vi "Compute SHA256 (byte array).vi"(10 "data in":u8[](array[numeric])) -> (2 "digest":u8[](array[numeric]) format="%02x")   [LabVIEW 2013, in "NI_SHA-256(2013).lvlib"]
doc: "Feed one final data buffer to the hash function, compute the message digest, and reset the hash function state."
uses:
  NI_SHA-256(2013).lvlib
  NI_SHA-256.lvclass
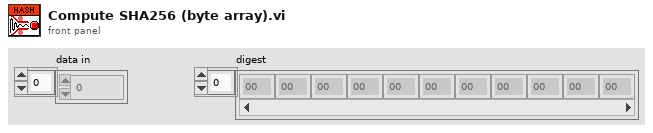
[diagram p1: front panel]
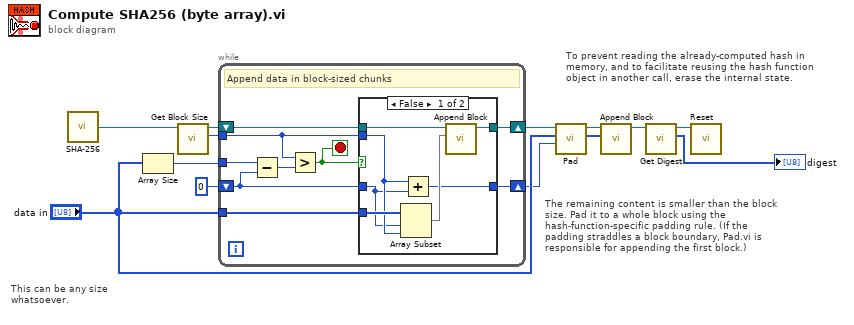
[diagram p0: block diagram]
diagram:
  # "To prevent reading the already-computed hash in memory, and to facilitate reusing the hash function object in another call, erase the internal state."
  # "The remaining content is smaller than the block size. Pad it to a whole block using the hash-function-specific padding rule. (If the padding straddles a block boundary, Pad.vi is responsible for appending the first block.)"
  # "This can be any size whatsoever."
  n1 = call "SHA-256.vi"() -> ("Hash Function out"=w1:refnum<class "NI_SHA-256.lvclass">)
  n2 = Array Size(array="data in") -> (size(s)=w7:i32)
  n3 = call "Get Block Size.vi"("Hash Function in"=w1) -> ("block size (bytes)"=w9:i32, "Hash Function out"=w11:refnum<class "NI_SHA-256.lvclass">)  [unwired: 9 in]
  n4 = while {
    shift-right: [w15] -> w8
    shift-left: w11 -> [w21]
    tunnel: w9 -> [w17]
    tunnel: "data in" -> [w18]
    tunnel: w7 -> [w22]
    shift-right: [w19] -> w5
    shift-left: 0 ("size(s)") -> [w20]
    stop <- w16 stop-if-true
    # "Append data in block-sized chunks"
    n5 = Subtract(x=w22, y=w20) -> (x-y=w14:i32)
    n6 = Greater?(x=w17, y=w14) -> (0:w16:bool)
    n7 = case shown="False" w16 {
      tunnel: w21 -> [w28 w31]
      tunnel: [w27 w31] -> w15
      tunnel: w20 -> [w24 w30]
      tunnel: [w23 w30] -> w19
      tunnel: w18 -> [w29 _]
      tunnel: w17 -> [w25 _]
      frame False {
        n8 = Array Subset(array=w29, index=w24, length=w25) -> (w26:u8[])
        n9 = Add(x=w25, y=w24) -> (x+y=w23:i32)
        n10 = call "Append Block.vi"("block in"=w26, "Hash Function in"=w28) -> ("Hash Function out"=w27:refnum<class "NI_SHA-256.lvclass">)  [unwired: 9 in]
      }
      frame True {
      }
    }
  }
  n11 = call "Pad.vi"("size"=w5, "data"="data in", "Hash Function in"=w8) -> ("padded block"=w3:u8[], "Hash Function out"=w4:refnum<class "NI_SHA-256.lvclass">)  [unwired: 7 in]
  n12 = call "Append Block.vi"("block in"=w3, "Hash Function in"=w4) -> ("Hash Function out"=w2:refnum<class "NI_SHA-256.lvclass">)  [unwired: 9 in]
  n13 = call "Get Digest.vi"("Hash Function in"=w2) -> ("Digest"=→"digest":u8[], "Hash Function out"=w6:refnum<class "NI_SHA-256.lvclass">)  [unwired: 9 in]
  n14 = call "Reset.vi"("Hash Function in"=w6) -> ()  [unwired: 10 in, 1 out]
